vi "Decide if iteration successful.vi"(8 "error in (no error)":errorcluster, 11 "RSA in":refnum<class "RSA.lvclass">) -> (0 "error out":errorcluster, 3 "RSA out":refnum<class "RSA.lvclass">)   [LabVIEW 2012, in "RSA.lvclass"]
uses:
  RSA.lvclass
  RSA.lvclass/RSA.ctl
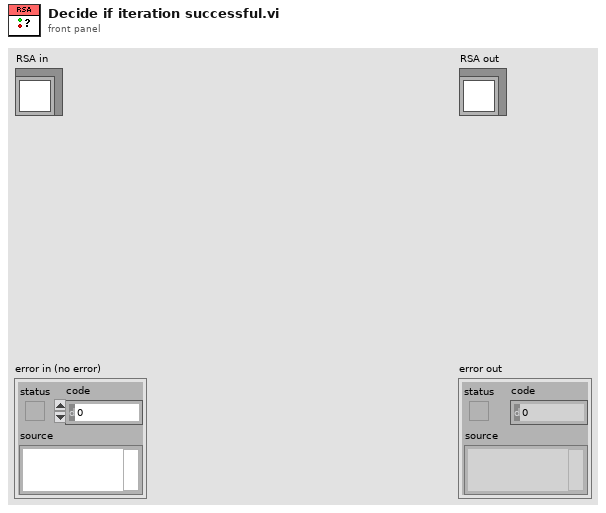
[diagram p1: front panel]
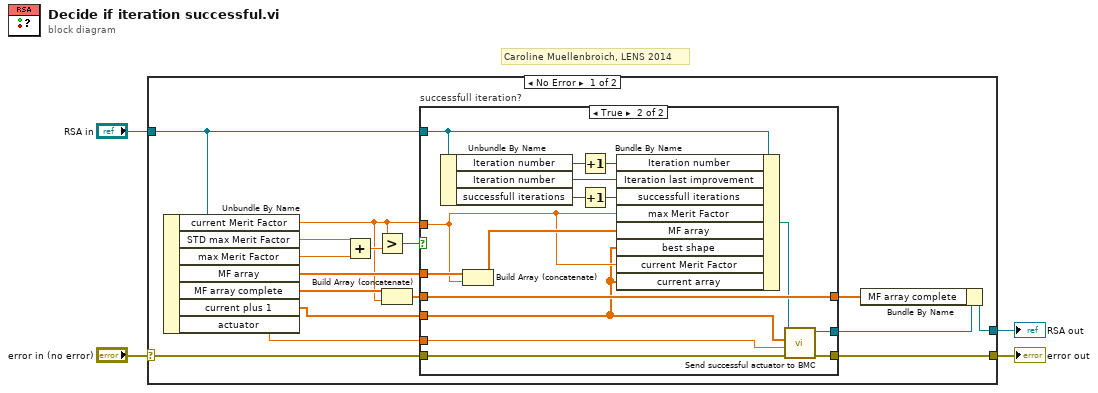
[diagram p0: block diagram]
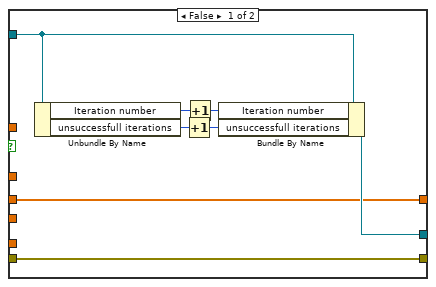
[diagram p2: hidden frame]
diagram:
  # "Caroline Muellenbroich, LENS 2014"
  n1 = case shown="No Error" "error in (no error)" {
    selector: "error in (no error)" -> [w12 w46]
    tunnel: [w9 w46] -> w3
    tunnel: [w16 w45] -> w1
    tunnel: "RSA in" -> [w17 w45]
    frame No Error {
      n2 = Unbundle By Name(w17) -> ("current Merit Factor"=w7:dbl, "STD max Merit Factor"=w20:dbl, "max Merit Factor"=w8:dbl, "MF array"=w14:dbl[], "MF array complete"=w13:dbl[], "current plus 1"=w6:dbl[], "actuator"=w5:dbl)
      n3 = Add(x=w20, y=w8) -> (x+y=w19:dbl)
      n4 = Greater?(x=w7, y=w19) -> (0:w18:bool)
      n5 = Build Array (concatenate)(w13, w7) -> (w11:dbl[])
      n6 = case "successfull iteration?" shown="True" w18 {
        tunnel: w17 -> [w26 w43]
        tunnel: [w25 w37] -> w15
        tunnel: w7 -> [_ w38]
        tunnel: w14 -> [_ w41]
        tunnel: w5 -> [_ w33]
        tunnel: w12 -> [w23 w34]
        tunnel: w11 -> [w24 w39]
        tunnel: [w24 w39] -> w10
        tunnel: [w23 w36] -> w9
        tunnel: w6 -> [_ w32]
        frame False {
          n7 = Unbundle By Name(w26) -> ("Iteration number"=w22:i32, "unsuccessfull iterations"=w28:i32)
          n8 = Increment(x=w28) -> (x+1=w27:i32)
          n9 = Increment(x=w22) -> (x+1=w21:i32)
          n10 = Bundle By Name(cluster=w26, "Iteration number"=w21, "unsuccessfull iterations"=w27) -> (w25:refnum<class "RSA.lvclass">)
        }
        frame True {
          n11 = Unbundle By Name(w43) -> ("Iteration number"=w29:i32, "Iteration number"=w42:i32, "successfull iterations"=w44:i32)
          n12 = Build Array (concatenate)(w41, w38) -> (w40:dbl[])
          n13 = Increment(x=w29) -> (x+1=w30:i32)
          n14 = Increment(x=w44) -> (x+1=w31:i32)
          n15 = Bundle By Name(cluster=w43, "Iteration number"=w30, "Iteration last improvement"=w42, "successfull iterations"=w31, "max Merit Factor"=w38, "MF array"=w40, "best shape"=w32, "current Merit Factor"=w38, "current array"=w32) -> (w35:refnum<class "RSA.lvclass">)
          n16 = call-dynamic "Send successful actuator to BMC.vi"("error in (no error)"=w34, "actuator in"=w33, "current plus 1 in"=w32, "RSA in"=w35) -> ("error out"=w36:errorcluster, "RSA out"=w37:refnum<class "RSA.lvclass">)  [unwired: 6 in]
        }
      }
      n17 = Bundle By Name(cluster=w15, "MF array complete"=w10) -> (w16:refnum<class "RSA.lvclass">)
    }
    frame Error {
    }
  }
  "error out" <- w3
  "RSA out" <- w1
